vi "IsItScratch.vi"(11 "Template":string) -> (3 "ScratchPad?":bool)   [LabVIEW 2022 SP3]
uses:
  Mic/Mic_Global.vi
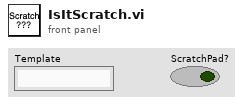
[diagram p1: front panel]
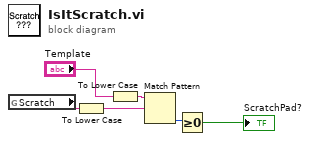
[diagram p0: block diagram]
diagram:
  n1 = global read "Mic_Global.vi" "Scratch"() -> (w2:string)
  n2 = To Lower Case(string=w2) -> (all lower case string=w6:string)
  n3 = To Lower Case(string="Template") -> (all lower case string=w5:string)
  n4 = Match Pattern(string=w5, regular expression=w6) -> (offset past match=w4:i32)  [unwired: 1 in, 3 out]
  n5 = Greater Or Equal To 0?(x=w4) -> (x >= 0?=→"ScratchPad?":bool)
